vi "Reverse_Norm.vi"(9 "Min":dbl, 10 "Max":dbl, 11 "Norm Value":dbl) -> (3 "Original Value":dbl)   [LabVIEW 2020]
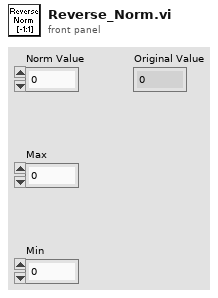
[diagram p1: front panel]
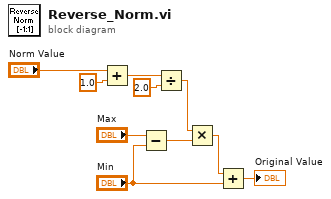
[diagram p0: block diagram]
diagram:
  n1 = Add(x="Norm Value", y=1.0) -> (x+y=w3:dbl)
  n2 = Subtract(x="Max", y="Min") -> (x-y=w6:dbl)
  n3 = Divide(x=w3, y=2.0) -> (x/y=w5:dbl)
  n4 = Multiply(x=w5, y=w6) -> (x*y=w8:dbl)
  n5 = Add(x=w8, y="Min") -> (x+y=→"Original Value":dbl)
